vi "SendMessage.vi"(2 "CmdArray":string="\u0000\u0003", 3 "receiver process":string="CueCmd", 4 "receiver host":string="169.254.48.3", 5 "receiver port (0)":u16=6378) -> (0 "error out":errorcluster)   [LabVIEW 2018]
uses:
  Target/CueState.ctl
  <vilib>/NI/AMC/Create Single Message.vi
  <vilib>/NI/AMC/Update Message Routing Info.vi
  <vilib>/NI/AMC/Send Message.vi
  <vilib>/NI/AMC/AMC.lvlib
panel:
  in  "message name":string="Cmd"
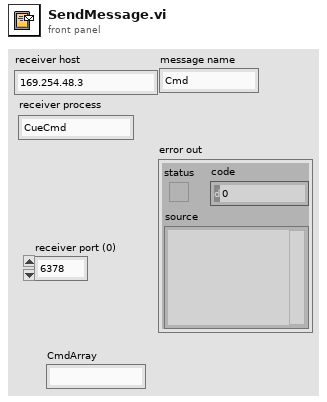
[diagram p1: front panel]
types:
  T1 = typedef "CueState.ctl" = enum16{"NetListen", "NetTalk", "Start", "Run", "Pause", "Unpause", "Skip wait", "Abort", "Finish"}
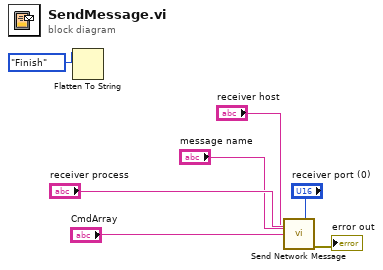
[diagram p0: block diagram]
diagram:
  n1 = Flatten To String(anything=CueState."Finish" ("Enum")) -> ()  [unwired: 3 in, 3 out]
  n2 = call <vilib>:"Send Network Message.vi"("receiver process"="receiver process", "receiver host"="receiver host", "receiver port (0)"="receiver port (0)", "message name"="message name", "message value"="CmdArray") -> ("error out"=→"error out":errorcluster)  [unwired: 8 in, 2 out]
